vi "Fix Lockin Parameters.vi"() -> ()   [LabVIEW 2024]
uses:
  NHMFL_Core/Libraries/SoftwareLockin/Lockin Parameters.ctl
panel:
  in  "Dest.  group name":string="p"
  in  "Dest.  channel name":string="Voltage"
  in  "Destination file path":path
  out "Output File Path":path
  in  "Cancel Button":bool
  out "found":bool
  in  "Save Button":bool
  in  "Lockin parameters":T1 {"DDS clock" format="%_17pHz"; "DDS modulus" format="0x%x (%d)"; "Phase" format="%#_gdeg"; "Frequency" format="%_17pHz"}
  out "Error Out":errorcluster
  in  "Error In":errorcluster
  in  "Source group name":string="p"
  in  "Source channel name":string="Voltage"
  in  "Source file path":path
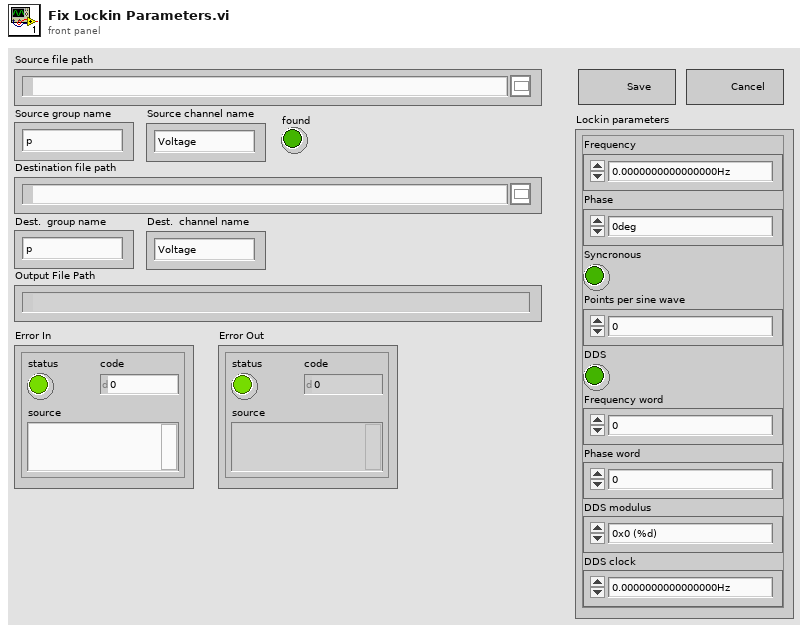
[diagram p1: front panel]
types:
  T1 = typedef "Lockin Parameters.ctl" = cluster{"Frequency":dbl, "Phase":dbl, "Syncronous":bool, "Points per sine wave":i32, "DDS":bool, "Frequency word":u32, "Phase word":u32, "DDS modulus":i64, "DDS clock":dbl}
  T2 = enum16{"open", "open or create", "create or replace", "create", "open (read-only)"}
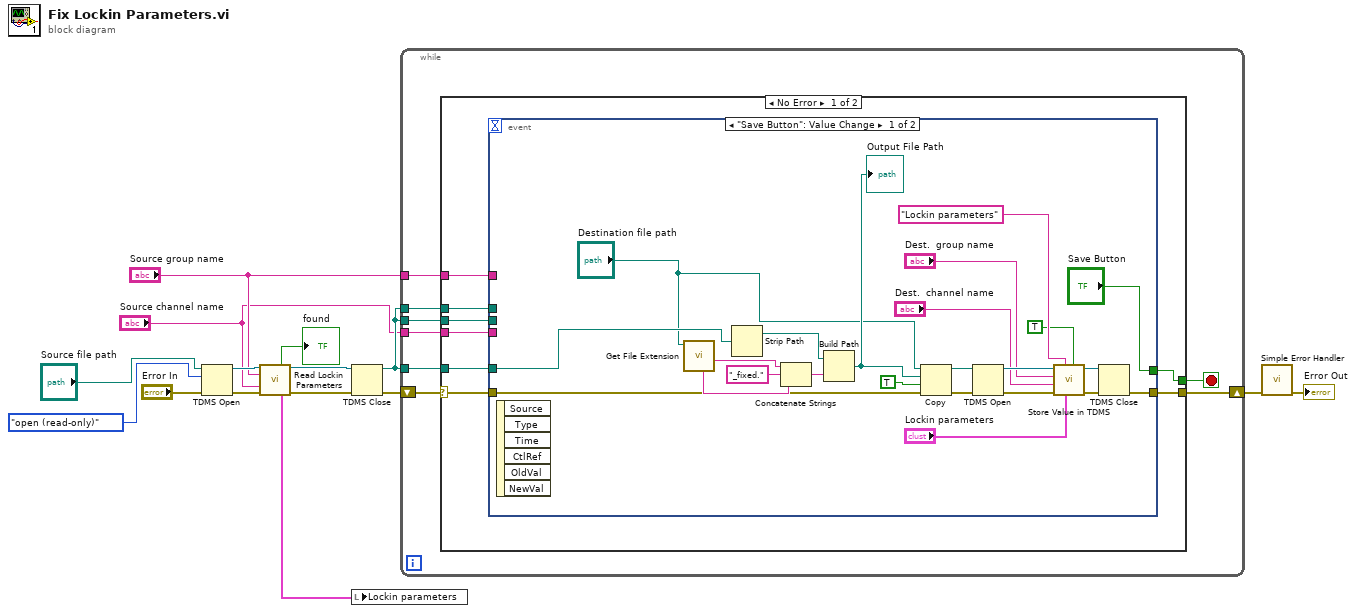
[diagram p0: block diagram]
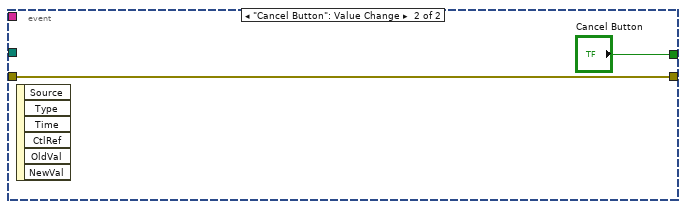
[diagram p2: hidden frame]
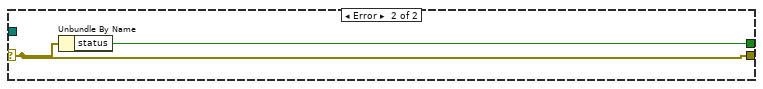
[diagram p3: hidden frame]
diagram:
  n1 = TDMS Open(8:"Error In", 10:T2."open (read-only)" ("operation (0:open)"), 11:"Source file path") -> (0:w9:errorcluster, 3:w10:refnum<k34>)  [unwired: 4 in]
  n2 = call "Read Lockin Parameters.vi"("tdms file"=w10, "group name in"="Source group name", "Channel name"="Source channel name", "Error In"=w9) -> ("found"=→"found":bool, "tdms file out"=w13:refnum<k34>, "Lockin parameters out"=w8:T1, "Error Out"=w12:errorcluster)  [unwired: 5 in, 3 out]
  n3 = TDMS Close(8:w12, 11:w13) -> (0:w6:errorcluster, 3:w4:path)
  n4 = local write "Lockin parameters"(w8) -> ()
  n5 = while {
    shift-right: [w21] -> w5
    shift-left: w6 -> [w22]
    tunnel: w4 -> [w20]
    tunnel: w4 -> [w19]
    tunnel: w4 -> [w18]
    tunnel: "Source group name" -> [w17]
    tunnel: "Source channel name" -> [w16]
    stop <- w23 stop-if-true
    n6 = case shown="No Error" w22 {
      selector: w22 -> [w30 w57]
      tunnel: [w31 w58] -> w23
      tunnel: [w29 w57] -> w21
      tunnel: w20 -> [w28 _]
      tunnel: w19 -> [w27 _]
      tunnel: w18 -> [w26 _]
      tunnel: w17 -> [w25 _]
      tunnel: w16 -> [w24 _]
      frame No Error {
        n7 = event shown="[0] \"Save Button\": Value Change" {
          selector: _ -> [_ _]
          dyn-events: _ -> [_ _]
          timeout: _ -> [_ _]
          tunnel: ["Save Button" "Cancel Button"] -> w31
          tunnel: [w38 w55] -> w29
          tunnel: w30 -> [w46 w55]
          tunnel: w28 -> [_ _]
          tunnel: w27 -> [_ _]
          tunnel: w26 -> [w48 _]
          tunnel: w25 -> [_ _]
          tunnel: w24 -> [_ _]
          event "Save Button": Value Change {
            n8 = event-data() -> ()  [unwired: 1 in, 6 out]
            n9 = call <vilib>:"Get File Extension.vi"("file"="Destination file path") -> ("filename without extension"=w50:string, "unmodified file extension"=w53:string)  [unwired: 6 in, 3 out]
            n10 = Strip Path(path=w48) -> (stripped path=w52:path)  [unwired: 1 out]
            n11 = Concatenate Strings(w50, "_fixed." ("string"), w53) -> (w51:string)
            n12 = Build Path(base path=w52, name or relative path=w51) -> (appended path=w47:path)
            "Output File Path" <- w47
            n13 = Copy(8:w46, 9:TRUE ("overwrite (F)"), 10:w47, 11:"Destination file path") -> (0:w44:errorcluster, 3:w45:path)  [unwired: 1 in, 1 out]
            n14 = TDMS Open(8:w44, 11:w45) -> (0:w43:errorcluster, 3:w42:refnum<k34>)  [unwired: 5 in]
            n15 = call "Store Value in TDMS.vi"("Replace name with prefix (FALSE = append)"=TRUE, "Value"="Lockin parameters", "Prefix"="Lockin parameters", "Error In"=w43, "channel name"="Dest.  channel name", "group name"="Dest.  group name", "tdms file"=w42) -> ("Error Out"=w40:errorcluster, "tdms file out"=w39:refnum<k34>)  [unwired: 1 in, 2 out]
            n16 = TDMS Close(8:w40, 11:w39) -> (0:w38:errorcluster)  [unwired: 1 out]
          }
          event "Cancel Button": Value Change {
            n17 = event-data() -> ()  [unwired: 1 in, 6 out]
          }
        }
      }
      frame Error {
        n18 = Unbundle By Name(w57) -> ("status"=w58:bool)
      }
    }
  }
  n19 = call <vilib>:"Simple Error Handler.vi"("error in (no error)"=w5) -> ("error out"=→"Error Out":errorcluster)  [unwired: 4 in, 4 out]
